vi "LVIS_UpdateMeas.vi"(8 "Error In":errorcluster, 11 "MeasName":string) -> (0 "Error out":errorcluster, 3 "MeasInfo":T1)   [LabVIEW 2015]
doc: "Updates the Measurement info based on the LVIS_Settings file configuration values."
uses:
  Globals/LVIS_IsGlobal.vi
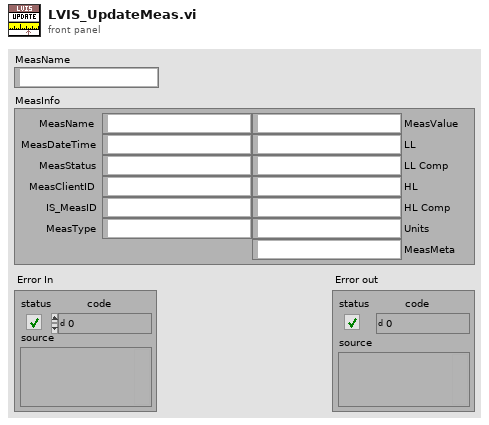
[diagram p1: front panel]
types:
  T1 = cluster{"MeasName":string, "MeasDateTime":string, "MeasStatus":string, "MeasClientID":string, "IS_MeasID":string, "MeasType":string, "MeasValue":string, "LL":string, "LL Comp":string, "HL":string, "HL Comp":string, "Units":string, "MeasMeta":string}
  T2 = cluster{"TestName":string, "TestDateTime":string, "TestStatus":string, "TestClientID":string, "IS_TestID":string, "TestMeta":string}
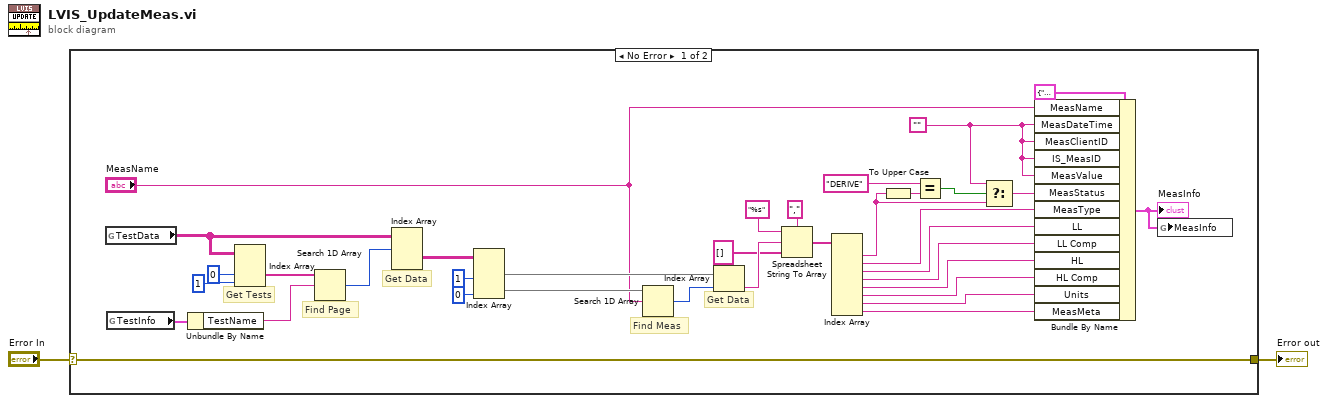
[diagram p0: block diagram]
diagram:
  n1 = case shown="No Error" "Error In" {
    selector: "Error In" -> [w29 w38]
    tunnel: [w29 w38] -> w1
    frame No Error {
      w6 = ""
      # "Get Data"
      # "Find Meas"
      # "Get Data"
      # "Find Page"
      # "Get Tests"
      n2 = global read "LVIS_IsGlobal.vi" "TestData"() -> (w35:string[][][])
      n3 = global read "LVIS_IsGlobal.vi" "TestInfo"() -> (w27:T2)
      n4 = Unbundle By Name(w27) -> ("TestName"=w26:string)
      n5 = Index Array(array=w35, index (dim 1)=0 ("disabled index (row)"), index (dim 2)=1 ("disabled index (col)")) -> (element=w36:string[])  [unwired: 1 in]
      n6 = Search 1D Array(1D array=w36, element=w26) -> (index of element=w34:i32)  [unwired: 1 in]
      n7 = Index Array(array=w35, index (dim 0)=w34) -> (element=w28:string[][])  [unwired: 2 in]
      n8 = Index Array(array=w28, index (col) #1=1 ("disabled index (col)"), index (col) #2=0 ("index (col)")) -> (element #1=w31:string[], element #2=w30:string[])  [unwired: 2 in]
      n9 = Search 1D Array(1D array=w30, element="MeasName") -> (index of element=w25:i32)  [unwired: 1 in]
      n10 = Index Array(array=w31, index=w25) -> (element=w23:string)
      n11 = Spreadsheet String To Array(delimiter (Tab)=",", format string="%s", spreadsheet string=w23, array type (2D Dbl)=string[] []) -> (array=w21:string[])
      n12 = Index Array(array=w21) -> (element #1=w8:string, element #2=w11:string, element #3=w12:string, element #4=w13:string, element #5=w14:string, element #6=w15:string, element #7=w16:string, element #8=w17:string)  [unwired: 8 in]
      n13 = To Upper Case(1:w8) -> (0:w3:string)
      n14 = Equal?(x="DERIVE", y=w3) -> (x = y?=w9:bool)
      n15 = Select(t=w6, s=w9, f=w8) -> (s? t:f=w7:string)
      n16 = Bundle By Name(cluster=T1 {"MeasName"="", "MeasDateTime"="", "MeasStatus"="", "MeasClientID"="", "IS_MeasID"="", "MeasType"="", "MeasValue"="", "LL"="", "LL Comp"="", "HL"="", "HL Comp"="", "Units"="", "MeasMeta"=""} ("MeasInfo"), "MeasName"="MeasName", "MeasDateTime"=w6, "MeasClientID"=w6, "IS_MeasID"=w6, "MeasValue"=w6, "MeasStatus"=w7, "MeasType"=w11, "LL"=w12, "LL Comp"=w13, "HL"=w14, "HL Comp"=w15, "Units"=w16, "MeasMeta"=w17) -> (w5:T1)
      "MeasInfo" <- w5
      n17 = global write "LVIS_IsGlobal.vi" "MeasInfo"(w5) -> ()
    }
    frame Error {
    }
  }
  "Error out" <- w1
